vi "Address Subscribe Message.vi"(9 "Return Priority (Normal)":T1=enum."Normal", 10 "Mediator Enqueuer":refnum<class "Message Enqueuer.lvclass">, 11 "Subscribe Msg In":refnum<class "Subscribe Msg.lvclass">) -> (3 "Subscribe Msg Out":refnum<class "Subscribe Msg.lvclass">)   [LabVIEW 2017, in "IMediator.lvlib" / "Subscribe Msg.lvclass"]
uses:
  <vilib>/gpm_packages/@cs/mva-core/Source/IMediator/IMediator Messages/Subscribe Msg/Subscribe Msg.lvclass
  C:/Program Files/National Instruments/LabVIEW 2017/vi.lib/gpm_packages/@cs/actor-framework-messages/Source/RoundTripMessage/RoundTripMessage.lvclass
  <vilib>/ActorFramework/Message Enqueuer/Message Enqueuer.lvclass
  <vilib>/ActorFramework/Message Enqueuer/Message Priority.ctl
  <vilib>/gpm_packages/@cs/actor-framework-messages/Source/RoundTripMessage/RoundTripMessage.lvclass/RoundTripMessage.ctl
  <vilib>/gpm_packages/@cs/actor-framework-messages/Source/RoundTripMessage/RoundTripMessage.lvclass
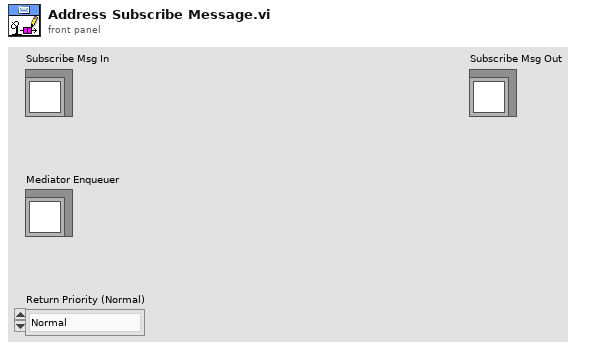
[diagram p1: front panel]
types:
  T1 = typedef "Actor Framework.lvlib/Message Enqueuer.lvclass/Message Priority.ctl" = enum16{"Low", "Normal", "High"}
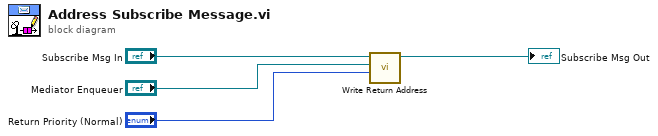
[diagram p0: block diagram]
diagram:
  n1 = call <vilib>:"Write Return Address.vi"("Return Priority (Normal)"="Return Priority (Normal)", "Return Enqueuer"="Mediator Enqueuer", "RoundTripMessage In"="Subscribe Msg In") -> ("RoundTripMessage Out"=→"Subscribe Msg Out":refnum<class "Subscribe Msg.lvclass">)  [unwired: 8 in]
